vi "Scanned.vi"() -> ()   [LabVIEW 2019]
panel:
  in  "Scanned":bool
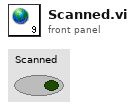
[diagram p1: front panel]
diagram:
